vi "Render.vi"(8 "error in (no error)":errorcluster, 11 "Alignment in":refnum<class "Alignment.lvclass">) -> (0 "error out":errorcluster, 3 "Alignment out":refnum<class "Alignment.lvclass">)   [LabVIEW 2021]
uses:
  Alignment.lvclass
  C:/GitHub/LvMarkdown/src/LvMarkdown/Markdown.lvclass
  C:/GitHub/LvMarkdown/src/LvMarkdown/Alignment/Alignment.lvclass
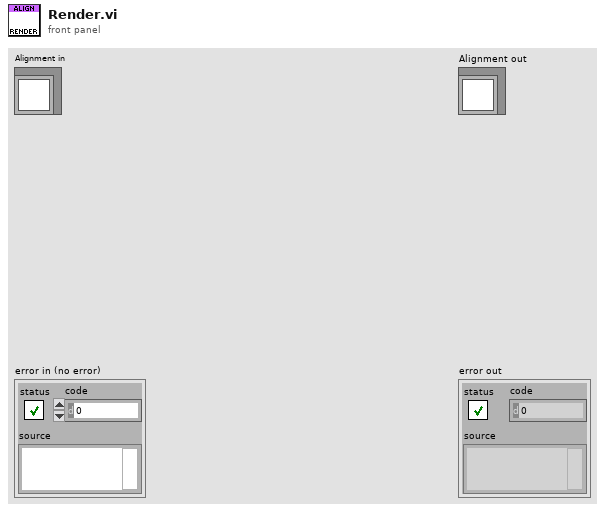
[diagram p1: front panel]
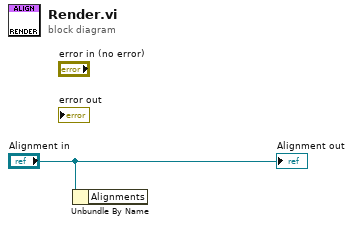
[diagram p0: block diagram]
diagram:
  n1 = Unbundle By Name("Alignment in") -> ()  [unwired: 1 out]
  "Alignment out" <- "Alignment in"
